vi "Set Log Folder.vi"(8 "error in (no error)":errorcluster, 10 "LogFolder":path, 11 "Node in":refnum<class "Node.lvclass">) -> (0 "error out":errorcluster, 3 "Node out":refnum<class "Node.lvclass">)   [LabVIEW 2020, in "VolatusConfig.lvlib" / "Node.lvclass"]
uses:
  Node.lvclass
  Node.lvclass/Node.ctl
  VolatusConfigElement/VolatusConfigElement.lvclass
  lv-cdm/CDM-Config/Config Element/Config Element.lvclass
  lv-cdm/CDM-Config/Value Type.ctl
  lv-cdm/CDM-Config/CDM-Config.lvlib
  C:/dev/lv20CE/relink/lv-volatus/VolatusConfig/VolatusConfigElement/VolatusConfigElement.lvclass
  C:/dev/lv20CE/relink/lv-volatus/VolatusConfig/Node/Node.lvclass
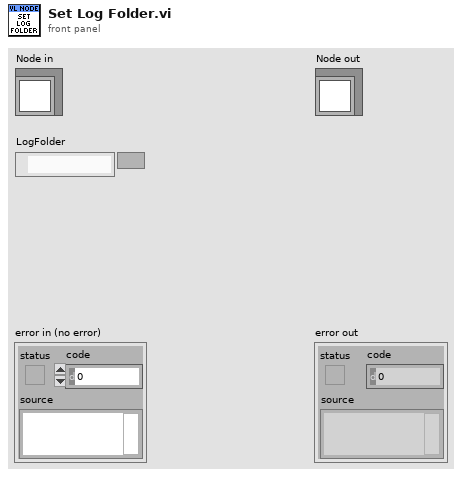
[diagram p1: front panel]
types:
  T1 = typedef "CDM-Config.lvlib/Value Type.ctl" = enum16{"String", "Number", "Bool", "Object", "Array"}
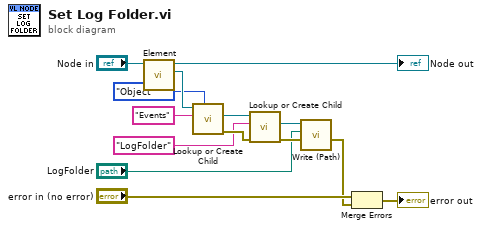
[diagram p0: block diagram]
diagram:
  n1 = call "Element.vi"("VolatusConfigElement in"="Node in") -> ("Element"=w11:refnum<class "Config Element.lvclass">, "VolatusConfigElement out"=→"Node out":refnum<class "Node.lvclass">)  [unwired: 9 in]
  n2 = call "Lookup or Create Child.vi"("Value Type (String)"=Value_Type."Object", "Name"="Events", "Config Element in"=w11) -> ("error out"=w7:errorcluster, "Child"=w8:refnum<class "Config Element.lvclass">)  [unwired: 5 in, 2 out]
  n3 = call "Lookup or Create Child.vi"("error in (no error)"=w7, "Name"="LogFolder", "Config Element in"=w8) -> ("error out"=w5:errorcluster, "Child"=w4:refnum<class "Config Element.lvclass">)  [unwired: 5 in, 2 out]
  n4 = call "Write (Path).vi"("error in (no error)"=w5, "Path Value"="LogFolder", "Config Element in"=w4) -> ("error out"=w1:errorcluster)  [unwired: 7 in, 1 out]
  n5 = Merge Errors("error in (no error)", w1) -> (→"error out":errorcluster)
